vi "TempMessung100AvgSub.vi"(0 "error out":errorcluster, 1 "address LockIn":string) -> (2 "error out 2":errorcluster, 3 "Numeric":dbl, 4 "mean":dbl)   [LabVIEW 2010]
uses:
  <vilib>/Analysis/NI_AALBase.lvlib
panel:
  out "Array":dbl[](array[numeric])
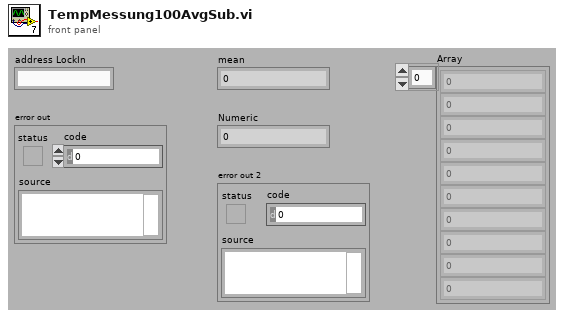
[diagram p1: front panel]
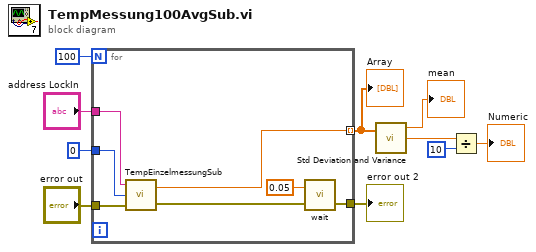
[diagram p0: block diagram]
diagram:
  n1 = for {
    N: 100 -> [_]
    tunnel: i16 0 ("mode (0)") -> [w16]
    tunnel: "address LockIn" -> [w17]
    tunnel: "error out" -> [w15]
    tunnel: [w11] -> w1 mode=indexing
    tunnel: [w12] -> w6
    n2 = call "TempEinzelmessungSub.vi"("error in"=w15, "mode (0)"=w16, "address string"=w17) -> ("error out"=w14:errorcluster, "Numeric"=w11:dbl)
    n3 = call "wait.vi"("error in"=w14, "Wartezeit in Sek"=0.05) -> ("error out"=w12:errorcluster)  [unwired: 1 in]
  }
  "error out 2" <- w6
  "Array" <- w1
  n4 = call <vilib>:"Std Deviation and Variance.vi"("X"=w1) -> ("mean"=→"mean":dbl, "standard deviation"=w2:dbl)  [unwired: 1 in, 1 out]
  n5 = Divide(x=w2, y=10) -> (x/y=→"Numeric":dbl)
